vi "tdms MC append shot numbers etc.vi"(7 "delete exising added channels":bool, 8 "error in (no error)":errorcluster, 9 "Scan info":T1, 10 "Bin Group in":i32[](array[numeric]), 11 "TDMS path":path) -> (0 "error out":errorcluster, 2 "Bin Group out":i32[](array[numeric]), 3 "TDMS path out":path)   [LabVIEW 2020]
uses:
  Scan info_typdef.ctl
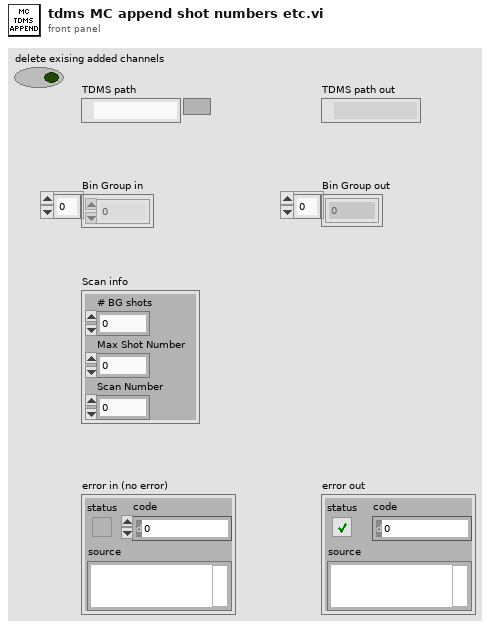
[diagram p1: front panel]
types:
  T1 = typedef "Scan info_typdef.ctl" = cluster{"# BG shots":i32, "Max Shot Number":i32, "Scan Number":i32}
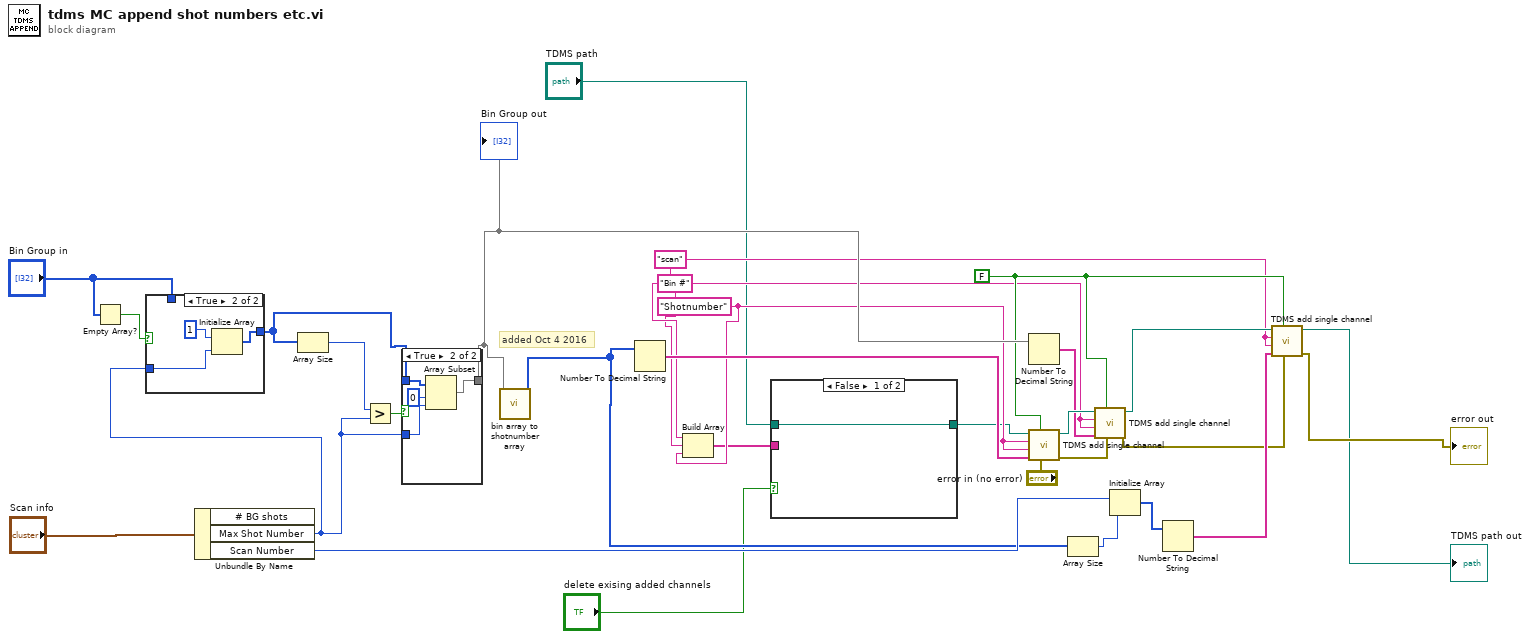
[diagram p0: block diagram]
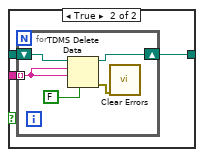
[diagram p2: hidden frame]
diagram:
  w7 = "scan" ("Device name")
  w6 = "Bin #" ("Device name")
  w5 = "Shotnumber" ("Device name")
  w13 = FALSE ("delete existing tdms file")
  # "added Oct 4 2016"
  n1 = Empty Array?(array="Bin Group in") -> (empty?=w27:bool)
  n2 = Unbundle By Name("Scan info") -> ("Max Shot Number"=w28:i32, "Scan Number"=w23:i32)  [unwired: 1 out]
  n3 = case shown="True" w27 {
    tunnel: w28 -> [_ w34]
    tunnel: [w31 w32] -> w30
    tunnel: "Bin Group in" -> [w31 _]
    frame False {
    }
    frame True {
      n4 = Initialize Array(1 ("Bin Group"), w34) -> (w32:i32[])
    }
  }
  n5 = Array Size(array=w30) -> (size(s)=w24:i32)
  n6 = Greater?(x=w24, y=w28) -> (0:w25:bool)
  n7 = case shown="True" w25 {
    tunnel: w30 -> [w35 w39]
    tunnel: [w35 w36] -> w26
    tunnel: w28 -> [_ w37]
    frame False {
    }
    frame True {
      n8 = Array Subset(array=w39, index=0, length=w37) -> (w36:i32[])
    }
  }
  "Bin Group out" <- w26
  n9 = call "bin array to shotnumber array.vi"("Bin Group"=w26) -> ("Shot numbers"=w19:i32[])  [unwired: 10 in]
  n10 = Number To Decimal String(number=w19) -> (decimal integer string=w12:string[])  [unwired: 1 in]
  n11 = Build Array(w7, w6, w5) -> (w4:string[])
  n12 = case shown="False" "delete exising added channels" {
    tunnel: w4 -> [_ w43]
    tunnel: "TDMS path" -> [w40 w42]
    tunnel: [w40 w41] -> w2
    frame False {
    }
    frame True {
      n13 = for {
        tunnel: w43 -> [w48] mode=indexing
        shift-right: [w46] -> w41
        shift-left: w42 -> [w47]
        n14 = TDMS Delete Data(6:FALSE ("keep empty group/channel? (T)"), 9:w48, 10:w48, 11:w47) -> (0:w45:errorcluster, 3:w46:path)  [unwired: 3 in]
        n15 = call <vilib>:"Clear Errors.vi"("error in (no error)"=w45) -> ()  [unwired: 5 in, 2 out]
      }
    }
  }
  n16 = Number To Decimal String(number=w26) -> (decimal integer string=w10:string[])  [unwired: 1 in]
  n17 = call "TDMS add single channel.vi"("error in"="error in (no error)", "delete existing tdms file"=w13, "Channel values"=w12, "Channel name"=w5, "Device name"=w5, "TDMS path"=w2) -> ("error out"=w9:errorcluster, "TDMS path out"=w11:path)  [unwired: 4 in]
  n18 = Array Size(array=w19) -> (size(s)=w20:i32)
  n19 = call "TDMS add single channel.vi"("error in"=w9, "delete existing tdms file"=w13, "Channel values"=w10, "Channel name"=w6, "Device name"=w6, "TDMS path"=w11) -> ("error out"=w16:errorcluster, "TDMS path out"=w14:path)  [unwired: 4 in]
  n20 = Initialize Array(w23, w20) -> (w21:i32[])
  n21 = Number To Decimal String(number=w21) -> (decimal integer string=w18:string[])  [unwired: 1 in]
  n22 = call "TDMS add single channel.vi"("error in"=w16, "delete existing tdms file"=w13, "Channel values"=w18, "Channel name"=w7, "Device name"=w7, "TDMS path"=w14) -> ("error out"=→"error out":errorcluster, "TDMS path out"=→"TDMS path out":path)  [unwired: 4 in]
